vi "perHandlemonochromator.vi"() -> ()   [LabVIEW 2011]
panel:
  out "peHandle":u32
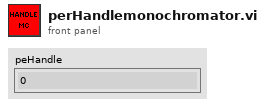
[diagram p1: front panel]
diagram:
